vi "Read Multiple Channels with Simple Header.vi"() -> ()   [LabVIEW 2012]
uses:
  <vilib>/Utility/file.llb/Read From Spreadsheet File (string).vi
panel:
  out "All Channels":dbl[][](graph)
  out "2-D Array of Strings":string[][](array[string])
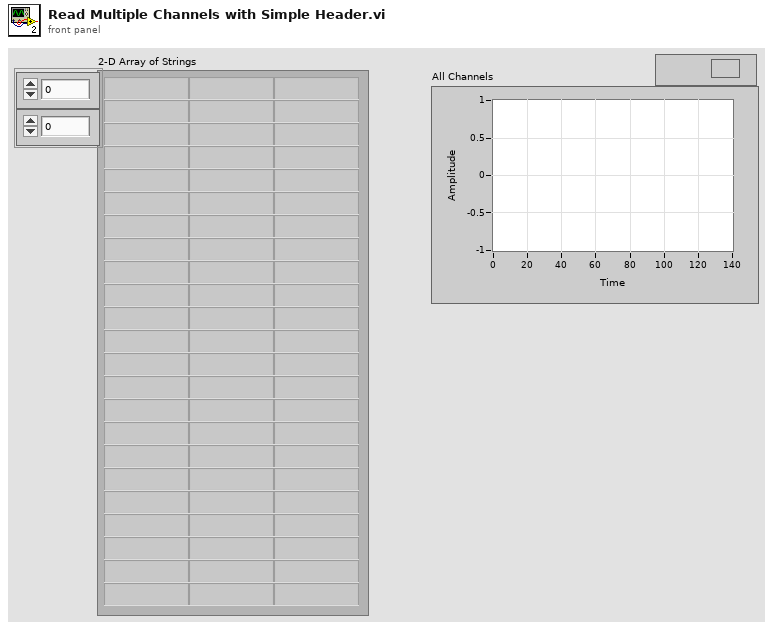
[diagram p1: front panel]
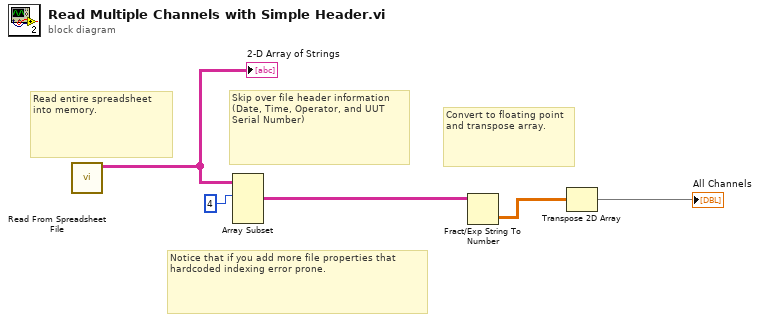
[diagram p0: block diagram]
diagram:
  # "Notice that if you add more file properties that hardcoded indexing error prone."
  # "Convert to floating point and transpose array."
  # "Skip over file header information (Date, Time, Operator, and UUT Serial Number)"
  # "Read entire spreadsheet into memory."
  n1 = call-poly <vilib>:"Read From Spreadsheet File.vi"() -> ("all rows"=w1:string[][])  [unwired: 7 in, 4 out]
  "2-D Array of Strings" <- w1
  n2 = Array Subset "Array Subset"(array=w1, index (row)=4 ("index")) -> (w3:string[][])  [unwired: 3 in]
  n3 = Fract/Exp String To Number(string=w3) -> (number=w5:dbl[][])  [unwired: 3 in, 1 out]
  n4 = Transpose 2D Array(2D array=w5) -> (transposed array=→"All Channels":dbl[][])
